vi "XLP80_Datalog_GetLogIndex.vi"(9 "CalcValueSize":i32) -> (0 "Unit Write":string[](array[string]), 1 "Name Write":string[](array[string]), 2 "Unit Read":string[](array[string]), 3 "Name Read":string[](array[string]), 4 "LogIndex":i32[](array[numeric]))   [LabVIEW 2021]
uses:
  XLP80_Globals/Globals_Settings_XLP80.vi
  XLP80_Globals/XLP80_Globals_Status.vi
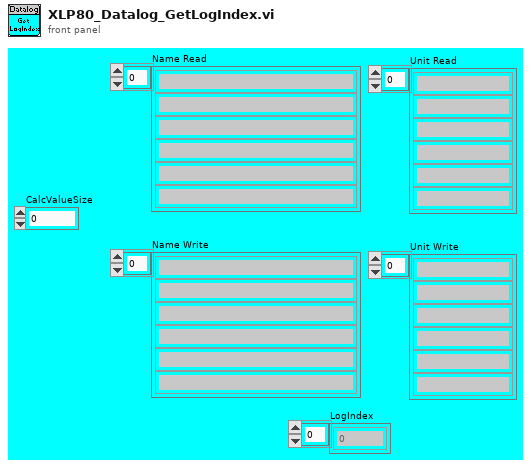
[diagram p1: front panel]
types:
  T1 = typedef "XLP80_Action_TDefEnumControl.ctl" = enum16{"Testmode_A", "Testmode_B"}
  T2 = typedef "XLP80_Datalog_TypeDefEnumLogselect.ctl" = enum16{"SMART.No.MaxCell [-]", "SMART.No.MinCell [-]", "SMART.U.S.AveCell [V]", "SMART.U.S.CVM [V]", "SMART.U.S.MaxCell [V]", "SMART.U.S.MinCell [V]"}
  T3 = cluster{"Signal Name":string[], "Description":string[], "Unit":string[], "Min":dbl[], "Max":dbl[], "TestmodeA":bool[], "LogEnable":bool[]}
  T4 = cluster{"Signal Name":string[], "Description":string[], "Unit":string[], "Default":dbl[], "Min":dbl[], "Max":dbl[], "TestmodeA":bool[], "LogEnable":bool[]}
  T5 = cluster{"Signal Name":string[], "Description":string[], "Unit":string[], "Min":dbl[], "Max":dbl[], "HV & Software":bool[], "Basis Funktion":bool[], "Power Management":bool[], "OperationMode":bool[], "Shutdown":bool[], "Alarm":bool[], "LogEnable":bool[]}
  T6 = cluster{"Signal Name":string[], "Description":string[], "Unit":string[], "Default":dbl[], "Min":dbl[], "Max":dbl[], "Preconditions":bool[], "HV & Software":bool[], "Basis Funktion":bool[], "Power Management":bool[], "OperationMode":bool[], "Shutdown":bool[], "Alarm":bool[], "LogEnable":bool[]}
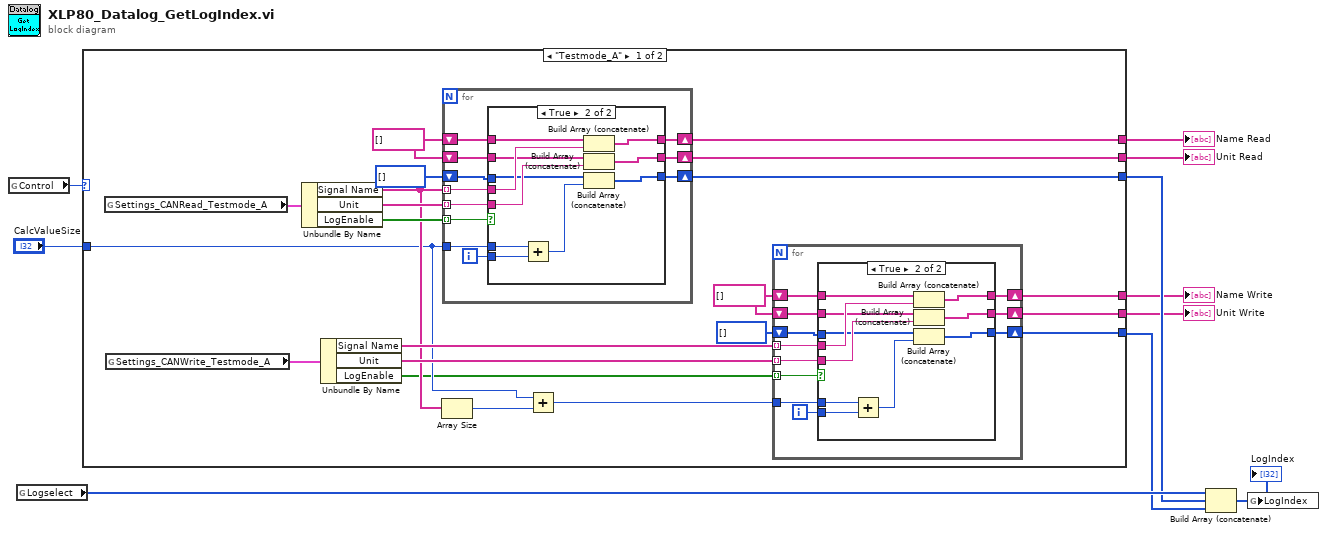
[diagram p0: block diagram]
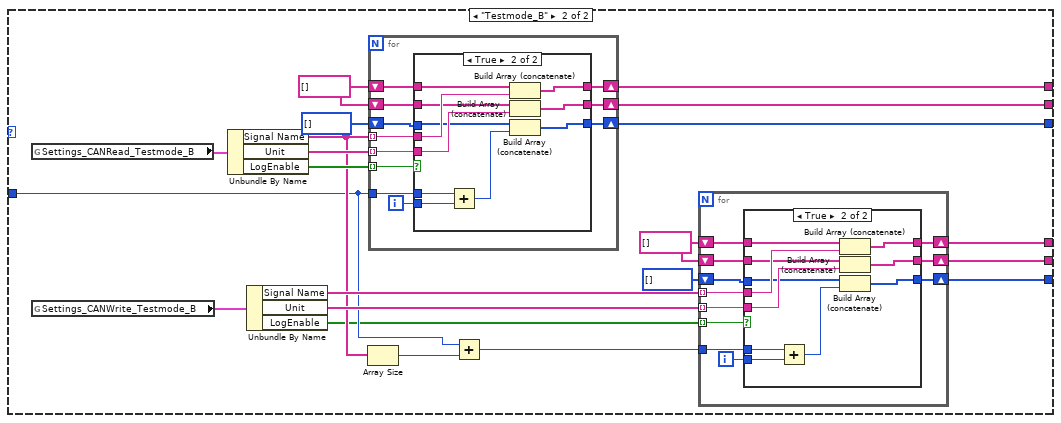
[diagram p4: hidden frame]
diagram:
  n1 = global read "XLP80_Globals_Status.vi" "Control"() -> (w10:T1)
  n2 = global read "Globals_Settings_XLP80.vi" "Logselect"() -> (w6:T2[])
  n3 = case shown="\"Testmode_A\"" w10 {
    tunnel: "CalcValueSize" -> [w16 w87]
    tunnel: [w26 w97] -> w8
    tunnel: [w25 w96] -> w7
    tunnel: [w23 w94] -> w5
    tunnel: [w14 w85] -> w3
    tunnel: [w12 w83] -> w2
    tunnel: [w11 w82] -> w1
    frame "Testmode_A" {
      w21 = string[] [] ("Signal Name")
      w27 = string[] [] ("Signal Name")
      n4 = global read "Globals_Settings_XLP80.vi" "Settings_CANRead_Testmode_A"() -> (w31:T3)
      n5 = global read "Globals_Settings_XLP80.vi" "Settings_CANWrite_Testmode_A"() -> (w30:T4)
      n6 = Unbundle By Name(w31) -> ("Signal Name"=w18:string[], "Unit"=w29:string[], "LogEnable"=w28:bool[])
      n7 = Unbundle By Name(w30) -> ("Signal Name"=w20:string[], "Unit"=w19:string[], "LogEnable"=w13:bool[])
      n8 = Array Size(array=w18) -> (size(s)=w17:i32)
      n9 = for {
        tunnel: w18 -> [w66] mode=indexing
        tunnel: w29 -> [w65] mode=indexing
        tunnel: w28 -> [w67] mode=indexing
        shift-right: [w62] -> w26
        shift-left: w27 -> [w64]
        shift-right: [w61] -> w25
        shift-left: w27 -> [w63]
        tunnel: w16 -> [w60]
        shift-right: [w58] -> w23
        shift-left: i32[] [] ("Signal Name") -> [w59]
        i -> [w57]
        n10 = case shown="True" w67 {
          tunnel: w66 -> [_ w80]
          tunnel: w65 -> [_ w77]
          tunnel: w64 -> [w70 w81]
          tunnel: w63 -> [w69 w78]
          tunnel: [w70 w79] -> w62
          tunnel: [w69 w76] -> w61
          tunnel: w60 -> [_ w74]
          tunnel: w59 -> [w68 w72]
          tunnel: [w68 w71] -> w58
          tunnel: w57 -> [_ w75]
          frame False {
          }
          frame True {
            n11 = Add(x=w74, y=w75) -> (x+y=w73:i32)
            n12 = Build Array (concatenate)(w81, w80) -> (w79:string[])
            n13 = Build Array (concatenate)(w78, w77) -> (w76:string[])
            n14 = Build Array (concatenate)(w72, w73) -> (w71:i32[])
          }
        }
      }
      n15 = Add(x=w16, y=w17) -> (x+y=w15:i32)
      n16 = for {
        tunnel: w20 -> [w41] mode=indexing
        tunnel: w19 -> [w40] mode=indexing
        tunnel: w13 -> [w42] mode=indexing
        shift-right: [w37] -> w12
        shift-left: w21 -> [w39]
        shift-right: [w36] -> w11
        shift-left: w21 -> [w38]
        tunnel: w15 -> [w35]
        shift-right: [w33] -> w14
        shift-left: i32[] [] ("Signal Name") -> [w34]
        i -> [w32]
        n17 = case shown="True" w42 {
          tunnel: w41 -> [_ w55]
          tunnel: w40 -> [_ w52]
          tunnel: w39 -> [w45 w56]
          tunnel: w38 -> [w44 w53]
          tunnel: [w45 w54] -> w37
          tunnel: [w44 w51] -> w36
          tunnel: w35 -> [_ w49]
          tunnel: w34 -> [w43 w47]
          tunnel: [w43 w46] -> w33
          tunnel: w32 -> [_ w50]
          frame False {
          }
          frame True {
            n18 = Add(x=w49, y=w50) -> (x+y=w48:i32)
            n19 = Build Array (concatenate)(w56, w55) -> (w54:string[])
            n20 = Build Array (concatenate)(w53, w52) -> (w51:string[])
            n21 = Build Array (concatenate)(w47, w48) -> (w46:i32[])
          }
        }
      }
    }
    frame "Testmode_B" {
      w92 = string[] [] ("Signal Name")
      w98 = string[] [] ("Signal Name")
      n22 = global read "Globals_Settings_XLP80.vi" "Settings_CANRead_Testmode_B"() -> (w102:T5)
      n23 = global read "Globals_Settings_XLP80.vi" "Settings_CANWrite_Testmode_B"() -> (w101:T6)
      n24 = Unbundle By Name(w102) -> ("Signal Name"=w89:string[], "Unit"=w100:string[], "LogEnable"=w99:bool[])
      n25 = Unbundle By Name(w101) -> ("Signal Name"=w91:string[], "Unit"=w90:string[], "LogEnable"=w84:bool[])
      n26 = Array Size(array=w89) -> (size(s)=w88:i32)
      n27 = for {
        tunnel: w89 -> [w137] mode=indexing
        tunnel: w100 -> [w136] mode=indexing
        tunnel: w99 -> [w138] mode=indexing
        shift-right: [w133] -> w97
        shift-left: w98 -> [w135]
        shift-right: [w132] -> w96
        shift-left: w98 -> [w134]
        tunnel: w87 -> [w131]
        shift-right: [w129] -> w94
        shift-left: i32[] [] ("Signal Name") -> [w130]
        i -> [w128]
        n28 = case shown="True" w138 {
          tunnel: w137 -> [_ w151]
          tunnel: w136 -> [_ w148]
          tunnel: w135 -> [w141 w152]
          tunnel: w134 -> [w140 w149]
          tunnel: [w141 w150] -> w133
          tunnel: [w140 w147] -> w132
          tunnel: w131 -> [_ w145]
          tunnel: w130 -> [w139 w143]
          tunnel: [w139 w142] -> w129
          tunnel: w128 -> [_ w146]
          frame False {
          }
          frame True {
            n29 = Add(x=w145, y=w146) -> (x+y=w144:i32)
            n30 = Build Array (concatenate)(w152, w151) -> (w150:string[])
            n31 = Build Array (concatenate)(w149, w148) -> (w147:string[])
            n32 = Build Array (concatenate)(w143, w144) -> (w142:i32[])
          }
        }
      }
      n33 = Add(x=w87, y=w88) -> (x+y=w86:i32)
      n34 = for {
        tunnel: w91 -> [w112] mode=indexing
        tunnel: w90 -> [w111] mode=indexing
        tunnel: w84 -> [w113] mode=indexing
        shift-right: [w108] -> w83
        shift-left: w92 -> [w110]
        shift-right: [w107] -> w82
        shift-left: w92 -> [w109]
        tunnel: w86 -> [w106]
        shift-right: [w104] -> w85
        shift-left: i32[] [] ("Signal Name") -> [w105]
        i -> [w103]
        n35 = case shown="True" w113 {
          tunnel: w112 -> [_ w126]
          tunnel: w111 -> [_ w123]
          tunnel: w110 -> [w116 w127]
          tunnel: w109 -> [w115 w124]
          tunnel: [w116 w125] -> w108
          tunnel: [w115 w122] -> w107
          tunnel: w106 -> [_ w120]
          tunnel: w105 -> [w114 w118]
          tunnel: [w114 w117] -> w104
          tunnel: w103 -> [_ w121]
          frame False {
          }
          frame True {
            n36 = Add(x=w120, y=w121) -> (x+y=w119:i32)
            n37 = Build Array (concatenate)(w127, w126) -> (w125:string[])
            n38 = Build Array (concatenate)(w124, w123) -> (w122:string[])
            n39 = Build Array (concatenate)(w118, w119) -> (w117:i32[])
          }
        }
      }
    }
  }
  "Name Read" <- w8
  "Unit Read" <- w7
  "Name Write" <- w2
  "Unit Write" <- w1
  n40 = Build Array (concatenate)(w6, w5, w3) -> (w4:i32[])
  "LogIndex" <- w4
  n41 = global write "XLP80_Globals_Status.vi" "LogIndex"(w4) -> ()
